vi "Query Application Status.vi"(0 "VISA resource name":refnum<visa-resource-name>, 11 "error in (no error)":errorcluster) -> (4 "VISA resource name out":refnum<visa-resource-name>, 6 "Application Status Out":T1(array[cluster]) {"Window" items=["Active", "Inactive", "Minimized", "Non"]; "Exists" items=["Exists", "Does not exist"]; "Status" items=["Current", "Run", "Idle", "Unload"]; "Application Name" items=["Signal Analyzer", "Spectrum Analyzer", "Config", "Signal Generator", "W-CDMA BS Meas", "WiMAX", "GSM", "HSDPA", "HSUPA", "TD-SCDMA", "LTE Uplink", "LTE Downlink"]}, 15 "error out":errorcluster)   [LabVIEW 2020, in "Anritsu Signal Analyzer Series.lvlib"]
doc: "Queries the status of the currently specified application."
uses:
  Anritsu Signal Analyzer Series.lvlib
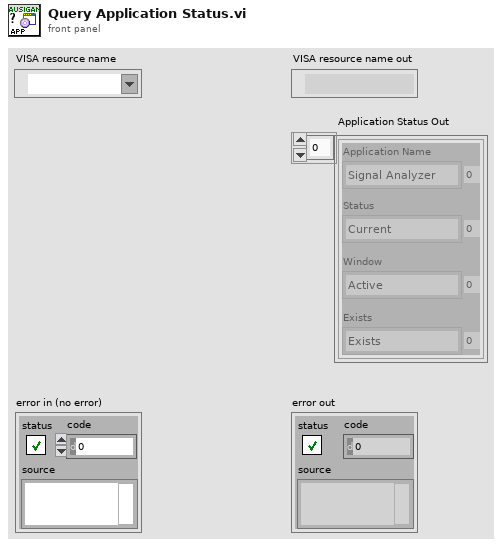
[diagram p1: front panel]
types:
  T1 = cluster{"Application Name":i32, "Status":i32, "Exists":i32, "Window":i32}[]
  T2 = cluster{"App (Signal Analyzer)":i32, "Status (Current)":i32, "Exists":i32, "Window (Active)":i32}
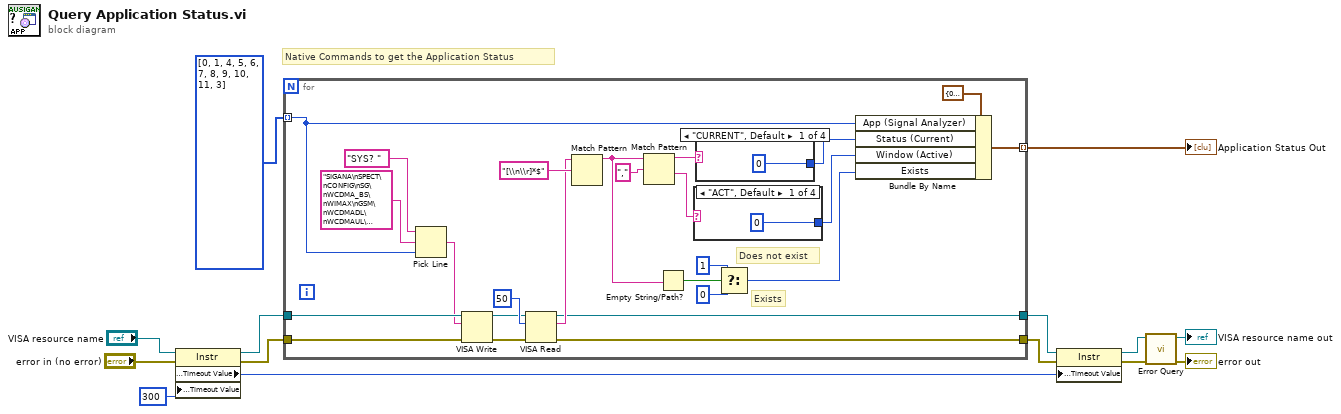
[diagram p0: block diagram]
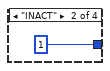
[diagram p2: hidden frame]
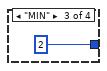
[diagram p3: hidden frame]
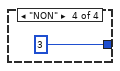
[diagram p4: hidden frame]
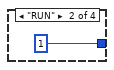
[diagram p5: hidden frame]
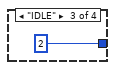
[diagram p6: hidden frame]
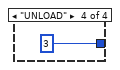
[diagram p7: hidden frame]
diagram:
  # "Native Commands to get the Application Status"
  n1 = property class="Instr"(reference="VISA resource name", error in="error in (no error)", "General Settings:Timeout Value"=u32 300) -> (reference out=w6:refnum<visa-resource-name>, error out=w5:errorcluster, "General Settings:Timeout Value"=w2:u32)
  n2 = for {
    tunnel: w6 -> [w28]
    tunnel: w5 -> [w27]
    tunnel: [w25] -> w3
    tunnel: [w26] -> w4
    tunnel: [w39] -> w8 mode=indexing
    tunnel: i32[] [0, 1, 4, 5, 6, 7, 8, 9, 10, 11, 3] -> [w15] mode=indexing
    # "Exists"
    # "Does not exist"
    n3 = Pick Line(string ("")="SYS? ", multi-line string="SIGANA\nSPECT\nCONFIG\nSG\nWCDMA_BS\nWIMAX\nGSM\nWCDMADL\nWCDMAUL\nTDSCDMA\n3GLTE_UL\n3GLTE_DL" ("文字列"), line index=w15) -> (output string=w18:string)
    n4 = VISA Write(VISA resource name=w28, write buffer=w18, error in (no error)=w27) -> (VISA resource name out=w29:refnum<visa-resource-name>, error out=w30:errorcluster)  [unwired: 1 out]
    n5 = VISA Read(VISA resource name=w29, byte count=u32 50 ("byte count (0)"), error in (no error)=w30) -> (VISA resource name out=w26:refnum<visa-resource-name>, read buffer=w32:string, error out=w25:errorcluster)  [unwired: 1 out]
    n6 = Match Pattern(string=w32, regular expression="[\\n\\r]*$") -> (before substring=w17:string)  [unwired: 1 in, 3 out]
    n7 = Match Pattern(string=w17, regular expression=",") -> (before substring=w35:string, after substring=w36:string)  [unwired: 1 in, 2 out]
    n8 = Empty String/Path?(string/path=w17) -> (empty?=w16:bool)
    n9 = case shown="\"ACT\", Default" w36 {
      tunnel: [0 ("Value out") 1 ("Value out") 2 ("Value out") 3 ("Value out")] -> w21
      frame "ACT", Default {
      }
      frame "INACT" {
      }
      frame "MIN" {
      }
      frame "NON" {
      }
    }
    n10 = case shown="\"CURRENT\", Default" w35 {
      tunnel: [0 ("Value out") 1 ("Value out") 2 ("Value out") 3 ("Value out")] -> w22
      frame "CURRENT", Default {
      }
      frame "RUN" {
      }
      frame "IDLE" {
      }
      frame "UNLOAD" {
      }
    }
    n11 = Select(t=1 ("Exists"), s=w16, f=0 ("Exists")) -> (s? t:f=w24:i32)
    n12 = Bundle By Name(cluster=T2 {"App (Signal Analyzer)"=0, "Status (Current)"=0, "Exists"=0, "Window (Active)"=0} ("Cluster"), "App (Signal Analyzer)"=w15, "Status (Current)"=w22, "Window (Active)"=w21, "Exists"=w24) -> (w39:T2)
  }
  "Application Status Out" <- w8
  n13 = property class="Instr"(reference=w4, error in=w3, "General Settings:Timeout Value"=w2) -> (reference out=w10:refnum<visa-resource-name>, error out=w9:errorcluster)
  n14 = call "Error Query.vi"("error in (no error)"=w9, "VISA resource name"=w10) -> ("error out"=→"error out":errorcluster, "VISA resource name out"=→"VISA resource name out":refnum<visa-resource-name>)  [unwired: 6 in, 2 out]
